vi "VI Task Manager.vi"() -> ()   [LabVIEW 2009]
panel:
  in  "?":bool
  in  "?":bool
  in  "?":bool
  in  "VIs":i32(listbox) caption="Top-level Running VIs"
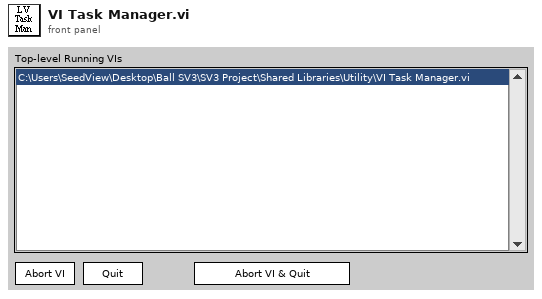
[diagram p1: front panel]
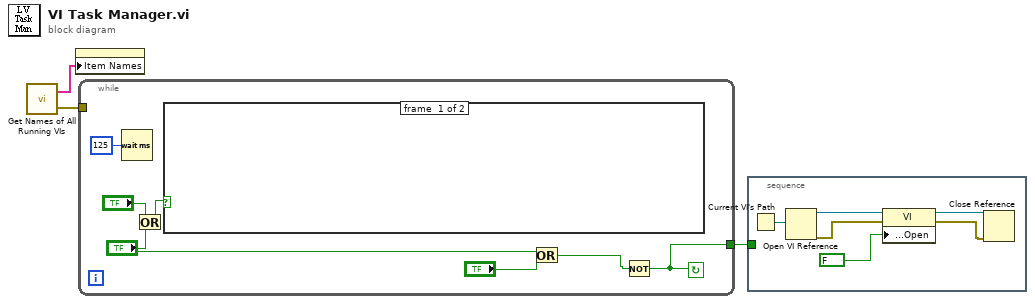
[diagram p0: block diagram]
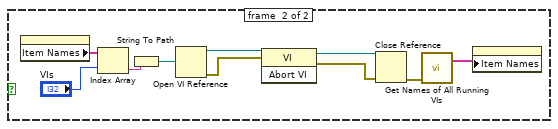
[diagram p2: hidden frame]
diagram:
  n1 = call "Get Names of All Running VIs.vi"() -> ("error out"=w1:errorcluster, "Item Names"=w2:string[])  [unwired: 2 in]
  n2 = property on="VIs" class="ListBox (strict)"("Item Names"=w2) -> ()  [unwired: 2 in, 2 out]
  n3 = while {
    tunnel: w1 -> [_]
    tunnel: [w9] -> w3
    stop <- w9 continue-if-true
    n4 = Wait (ms)(milliseconds to wait=u32 125) -> ()  [unwired: 1 out]
    n5 = Or(x="?", y="?") -> (x .or. y?=w5:bool)
    n6 = case shown="True" w5 {
      frame #0 {
      }
      frame #1 {
        n7 = property on="VIs" class="ListBox (strict)"() -> ("Item Names"=w20:string[])  [unwired: 2 in, 2 out]
        n8 = Index Array(array=w20, index="VIs") -> (element=w14:string)
        n9 = String To Path(string=w14) -> (path=w13:path)
        n10 = Open VI Reference(vi path=w13) -> (vi reference=w18:refnum<vi>, error out=w17:errorcluster)  [unwired: 5 in]
        n11 = invoke class="VI" method="Abort VI"(reference=w18, error in=w17) -> (reference out=w16:refnum<vi>, error out=w15:errorcluster)  [unwired: 1 in, 1 out]
        n12 = Close Reference(reference=w16, error in (no error)=w15) -> (error out=w12:errorcluster)
        n13 = call "Get Names of All Running VIs.vi"("error in (no error)"=w12) -> ("Item Names"=w11:string[])  [unwired: 1 in, 1 out]
        n14 = property on="VIs" class="ListBox (strict)"("Item Names"=w11) -> ()  [unwired: 2 in, 2 out]
      }
    }
    n15 = Or(x="?", y="?") -> (x .or. y?=w7:bool)
    n16 = Not(x=w7) -> (.not. x?=w9:bool)
  }
  n17 = stacked-sequence {
    tunnel: w3 -> [_]
    frame #0 {
      n18 = Current VI's Path() -> (path=w26:path)
      n19 = Open VI Reference(vi path=w26) -> (vi reference=w25:refnum<vi>, error out=w24:errorcluster)  [unwired: 5 in]
      n20 = property class="VI"(reference=w25, error in=w24, "Front Panel Window:Open"=FALSE ("Front Panel.Open")) -> (reference out=w22:refnum<vi>, error out=w21:errorcluster)
      n21 = Close Reference(reference=w22, error in (no error)=w21) -> ()  [unwired: 1 out]
    }
  }
